vi "ExecutionControlGlobal.vi"() -> ()   [LabVIEW 2013]
panel:
  out "Stop":bool
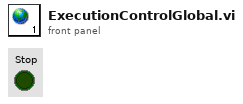
[diagram p1: front panel]
diagram:
